vi "FaulhaberV3-Ascii_V1.vi"() -> (1 "searchnames":string[](array[string]), 2 "ID":u32[](array[numeric]), 3 "Faulhaber Objects":T3(array[cluster]))   [LabVIEW 2011] (continued)
7\" dataType=\"0006\" accessType=\"ro\" PDOmapping=\"TPDO\" />\n\t\t\t\t\t</CANopenObject>\n\t\t\t\t\t<CANopenObject index=\"2316\" name=\"Reference encoder\" objectType=\"9\" subNumber=\"8\">\n\t\t\t\t\t\t<CANopenSubObject subIndex=\"00\" name=\"Number of entries\" objectType=\"7\" dataType=\"0005\" accessType=\"ro\" defaultValue=\"9\" PDOmapping=\"no\" />\n\t\t\t\t\t\t<CANopenSubObject subIndex=\"01\" name=\"Operation mode, index polarity\" objectType=\"7\" dataType=\"0006\" lowLimit=\"0\" highLimit=\"0x0107\" accessType=\"rw\" defaultValue=\"0x0\" PDOmapping=\"no\" objFlags=\"00020000\" />\n\t\t\t\t\t\t<CANopenSubObject subIndex=\"02\" name=\"IE resolution\" objectType=\"7\" dataType=\"0007\" lowLimit=\"0\" highLimit=\"4294967295\" accessType=\"rw\" defaultValue=\"2048\" PDOmapping=\"no\" objFlags=\"00020000\" />\n\t\t\t\t\t\t<CANopenSubObject subIndex=\"03\" name=\"Reference encoder position\" objectType=\"7\" dataType=\"0004\" accessType=\"ro\" PDOmapping=\"TPDO\" />\n\t\t\t\t\t\t<CANopenSubObject subIndex=\"04\" name=\"Gain  (numerator/divisor)\" objectType=\"7\" dataType=\"0004\" lowLimit=\"-2147483648\" highLimit=\"2147483647\" accessType=\"rw\" defaultValue=\"0x40004000\" PDOmapping=\"RPDO\" objFlags=\"00020000\" />\n\t\t\t\t\t\t<CANopenSubObject subIndex=\"05\" name=\"RefEnc scaled position\" objectType=\"7\" dataType=\"0004\" lowLimit=\"-2147483648\" highLimit=\"2147483647\" accessType=\"rw\" defaultValue=\"0\" PDOmapping=\"TPDO\" />\n\t\t\t\t\t\t<CANopenSubObject subIndex=\"08\" name=\"Reference encoder act speed\" objectType=\"7\" dataType=\"0004\" accessType=\"ro\" PDOmapping=\"TPDO\" />\n\t\t\t\t\t\t<CANopenSubObject subIndex=\"09\" name=\"Speed filter\" objectType=\"7\" dataType=\"0006\" lowLimit=\"0\" highLimit=\"65535\" accessType=\"rw\" defaultValue=\"10\" PDOmapping=\"TPDO\" objFlags=\"00020000\" />\n\t\t\t\t\t</CANopenObject>\n\t\t\t\t\t<CANopenObject index=\"2317\" name=\"PWM input\" objectType=\"9\" subNumber=\"8\">\n\t\t\t\t\t\t<CANopenSubObject subIndex=\"00\" name=\"Number of entries\" objectType=\"7\" dataType=\"0005\" accessType=\"ro\" defaultValue=\"7\" PDOmapping=\"no\" />\n\t\t\t\t\t\t<CANopenSubObject subIndex=\"01\" name=\"Digital input pin\" objectType=\"7\" dataType=\"0005\" PDOmapping=\"no\" objFlags=\"00020000\" uniqueIDRef=\"UID_PARAM_231701\" />\n\t\t\t\t\t\t<CANopenSubObject subIndex=\"02\" name=\"PWM input frequency\" objectType=\"7\" dataType=\"0007\" accessType=\"ro\" PDOmapping=\"TPDO\" objFlags=\"00020000\" />\n\t\t\t\t\t\t<CANopenSubObject subIndex=\"03\" name=\"Duty cycle raw value\" objectType=\"7\" dataType=\"0003\" accessType=\"ro\" PDOmapping=\"TPDO\" objFlags=\"00020000\" />\n\t\t\t\t\t\t<CANopenSubObject subIndex=\"04\" name=\"Duty cycle  gain (numerator/divisor)\" objectType=\"7\" dataType=\"0007\" lowLimit=\"0\" highLimit=\"4294967295\" accessType=\"rw\" defaultValue=\"0x7FFF8000\" PDOmapping=\"no\" objFlags=\"00020000\" />\n\t\t\t\t\t\t<CANopenSubObject subIndex=\"05\" name=\"Duty cycle offset\" objectType=\"7\" dataType=\"0003\" lowLimit=\"-32768\" highLimit=\"32767\" accessType=\"rw\" defaultValue=\"0\" PDOmapping=\"RPDO\" objFlags=\"00020000\" />\n\t\t\t\t\t\t<CANopenSubObject subIndex=\"06\" name=\"Duty cycle scaled value\" objectType=\"7\" dataType=\"0004\" accessType=\"ro\" PDOmapping=\"TPDO\" objFlags=\"00020000\" />\n\t\t\t\t\t\t<CANopenSubObject subIndex=\"07\" name=\"Resolution as encoder\" objectType=\"7\" dataType=\"0003\" lowLimit=\"-32768\" highLimit=\"32767\" accessType=\"rw\" defaultValue=\"1000\" PDOmapping=\"no\" objFlags=\"00020000\" />\n\t\t\t\t\t</CANopenObject>\n\t\t\t\t\t<CANopenObject index=\"2318\" name=\"Hall configuration\" objectType=\"9\" subNumber=\"6\">\n\t\t\t\t\t\t<CANopenSubObject subIndex=\"00\" name=\"Number of entries\" objectType=\"7\" dataType=\"0005\" accessType=\"ro\" defaultValue=\"5\" PDOmapping=\"no\" />\n\t\t\t\t\t\t<CANopenSubObject subIndex=\"01\" name=\"Hall sensor type\" objectType=\"7\" dataType=\"0005\" highLimit=\"0x83\" accessType=\"ro\" PDOmapping=\"no\" objFlags=\"00030000\" />\n\t\t\t\t\t\t<CANopenSubObject subIndex=\"02\" name=\"Enable adaptation\" objectType=\"7\" dataType=\"0005\" lowLimit=\"0\" highLimit=\"255\" accessType=\"rw\" defaultValue=\"0\" PDOmapping=\"no\" objFlags=\"00020000\" />\n\t\t\t\t\t\t<CANopenSubObject subIndex=\"03\" name=\"Adaptation threshold speed\" objectType=\"7\" dataType=\"0007\" lowLimit=\"0\" highLimit=\"4294967295\" accessType=\"rw\" defaultValue=\"1000\" PDOmapping=\"no\" objFlags=\"00020000\" />\n\t\t\t\t\t\t<CANopenSubObject subIndex=\"04\" name=\"Digital hall settings of Non-Faulhaber motors\" objectType=\"7\" dataType=\"0005\" lowLimit=\"0\" highLimit=\"0x81\" accessType=\"rw\" defaultValue=\"0x0\" PDOmapping=\"no\" objFlags=\"00020000\" />\n\t\t\t\t\t\t<CANopenSubObject subIndex=\"05\" name=\"Hall filter configuration\" objectType=\"7\" dataType=\"0005\" lowLimit=\"0\" highLimit=\"0x03\" accessType=\"rw\" defaultValue=\"0x0\" PDOmapping=\"no\" objFlags=\"00020000\" />\n\t\t\t\t\t</CANopenObject>\n\t\t\t\t\t<CANopenObject index=\"2319\" name=\"Reduction ratio, external position encoder\" objectType=\"8\" subNumber=\"3\">\n\t\t\t\t\t\t<CANopenSubObject subIndex=\"00\" name=\"Number of entries\" objectType=\"7\" dataType=\"0005\" accessType=\"ro\" defaultValue=\"2\" PDOmapping=\"no\" />\n\t\t\t\t\t\t<CANopenSubObject subIndex=\"01\" name=\"Numerator\" objectType=\"7\" dataType=\"0007\" lowLimit=\"1\" highLimit=\"4294967295\" accessType=\"rw\" defaultValue=\"1\" PDOmapping=\"RPDO\" objFlags=\"00020000\" />\n\t\t\t\t\t\t<CANopenSubObject subIndex=\"02\" name=\"Divisor\" objectType=\"7\" dataType=\"0007\" lowLimit=\"1\" highLimit=\"4294967295\" accessType=\"rw\" defaultValue=\"1\" PDOmapping=\"RPDO\" objFlags=\"00020000\" />\n\t\t\t\t\t</CANopenObject>\n\t\t\t\t\t<CANopenObject index=\"231F\" name=\"231F_00\" objectType=\"8\" subNumber=\"16\">\n\t\t\t\t\t\t<CANopenSubObject subIndex=\"00\" name=\"Number of entries\" objectType=\"7\" dataType=\"0005\" accessType=\"ro\" defaultValue=\"15\" PDOmapping=\"no\" objFlags=\"00020003\" />\n\t\t\t\t\t\t<CANopenSubObject subIndex=\"01\" name=\"231F_01\" objectType=\"7\" dataType=\"0003\" accessType=\"ro\" PDOmapping=\"no\" objFlags=\"00020003\" />\n\t\t\t\t\t\t<CANopenSubObject subIndex=\"02\" name=\"231F_02\" objectType=\"7\" dataType=\"0003\" accessType=\"ro\" PDOmapping=\"no\" objFlags=\"00020003\" />\n\t\t\t\t\t\t<CANopenSubObject subIndex=\"03\" name=\"231F_03\" objectType=\"7\" dataType=\"0003\" accessType=\"ro\" PDOmapping=\"no\" objFlags=\"00020003\" />\n\t\t\t\t\t\t<CANopenSubObject subIndex=\"04\" name=\"231F_04\" objectType=\"7\" dataType=\"0003\" accessType=\"ro\" PDOmapping=\"no\" objFlags=\"00020003\" />\n\t\t\t\t\t\t<CANopenSubObject subIndex=\"05\" name=\"231F_05\" objectType=\"7\" dataType=\"0003\" accessType=\"ro\" PDOmapping=\"no\" objFlags=\"00020003\" />\n\t\t\t\t\t\t<CANopenSubObject subIndex=\"06\" name=\"231F_06\" objectType=\"7\" dataType=\"0003\" accessType=\"ro\" PDOmapping=\"no\" objFlags=\"00020003\" />\n\t\t\t\t\t\t<CANopenSubObject subIndex=\"07\" name=\"231F_07\" objectType=\"7\" dataType=\"0003\" accessType=\"ro\" PDOmapping=\"no\" objFlags=\"00020003\" />\n\t\t\t\t\t\t<CANopenSubObject subIndex=\"08\" name=\"231F_08\" objectType=\"7\" dataType=\"0003\" accessType=\"ro\" PDOmapping=\"no\" objFlags=\"00020003\" />\n\t\t\t\t\t\t<CANopenSubObject subIndex=\"09\" name=\"231F_09\" objectType=\"7\" dataType=\"0003\" accessType=\"ro\" PDOmapping=\"no\" objFlags=\"00020003\" />\n\t\t\t\t\t\t<CANopenSubObject subIndex=\"0A\" name=\"231F_0A\" objectType=\"7\" dataType=\"0003\" accessType=\"ro\" PDOmapping=\"no\" objFlags=\"00020003\" />\n\t\t\t\t\t\t<CANopenSubObject subIndex=\"0B\" name=\"231F_0B\" objectType=\"7\" dataType=\"0003\" accessType=\"ro\" PDOmapping=\"no\" objFlags=\"00020003\" />\n\t\t\t\t\t\t<CANopenSubObject subIndex=\"0C\" name=\"231F_0C\" objectType=\"7\" dataType=\"0003\" accessType=\"ro\" PDOmapping=\"no\" objFlags=\"00020003\" />\n\t\t\t\t\t\t<CANopenSubObject subIndex=\"0D\" name=\"231F_0D\" objectType=\"7\" dataType=\"0003\" accessType=\"ro\" PDOmapping=\"no\" objFlags=\"00020003\" />\n\t\t\t\t\t\t<CANopenSubObject subIndex=\"0E\" name=\"231F_0E\" objectType=\"7\" dataType=\"0003\" accessType=\"ro\" PDOmapping=\"no\" objFlags=\"00020003\" />\n\t\t\t\t\t\t<CANopenSubObject subIndex=\"0F\" name=\"231F_0F\" objectType=\"7\" dataType=\"0003\" accessType=\"ro\" PDOmapping=\"no\" objFlags=\"00020003\" />\n\t\t\t\t\t</CANopenObject>\n\t\t\t\t\t<CANopenObject index=\"2320\" name=\"Faulhaber error register\" objectType=\"7\" dataType=\"0006\" accessType=\"ro\" PDOmapping=\"TPDO\" />\n\t\t\t\t\t<CANopenObject index=\"2321\" name=\"Error mask\" objectType=\"8\" subNumber=\"8\">\n\t\t\t\t\t\t<CANopenSubObject subIndex=\"00\" name=\"Number of entries\" objectType=\"7\" dataType=\"0005\" accessType=\"ro\" defaultValue=\"7\" PDOmapping=\"no\" />\n\t\t\t\t\t\t<CANopenSubObject subIndex=\"01\" name=\"EMCY mask\" objectType=\"7\" dataType=\"0006\" lowLimit=\"0\" highLimit=\"65535\" accessType=\"rw\" defaultValue=\"0xFFFF\" PDOmapping=\"RPDO\" objFlags=\"00020000\" />\n\t\t\t\t\t\t<CANopenSubObject subIndex=\"02\" name=\"Fault mask\" objectType=\"7\" dataType=\"0006\" lowLimit=\"0\" highLimit=\"0xBFD3\" accessType=\"rw\" defaultValue=\"0x0000\" PDOmapping=\"RPDO\" objFlags=\"00020000\" />\n\t\t\t\t\t\t<CANopenSubObject subIndex=\"03\" name=\"Error out mask\" objectType=\"7\" dataType=\"0006\" lowLimit=\"0\" highLimit=\"65535\" accessType=\"rw\" defaultValue=\"0x0000\" PDOmapping=\"RPDO\" objFlags=\"00020000\" />\n\t\t\t\t\t\t<CANopenSubObject subIndex=\"04\" name=\"Disable voltage mask manufacturer\" objectType=\"7\" dataType=\"0006\" accessType=\"ro\" defaultValue=\"0x402C\" PDOmapping=\"no\" objFlags=\"00030000\" />\n\t\t\t\t\t\t<CANopenSubObject subIndex=\"05\" name=\"Disable voltage mask user\" objectType=\"7\" dataType=\"0006\" lowLimit=\"0\" highLimit=\"0xBFD3\" accessType=\"rw\" defaultValue=\"0x0000\" PDOmapping=\"RPDO\" objFlags=\"00020000\" />\n\t\t\t\t\t\t<CANopenSubObject subIndex=\"06\" name=\"Quick stop mask\" objectType=\"7\" dataType=\"0006\" lowLimit=\"0\" highLimit=\"0xBFD3\" accessType=\"rw\" defaultValue=\"0x0000\" PDOmapping=\"RPDO\" objFlags=\"00020000\" />\n\t\t\t\t\t\t<CANopenSubObject subIndex=\"07\" name=\"Error bit mask\" objectType=\"7\" dataType=\"0006\" lowLimit=\"0\" highLimit=\"65535\" accessType=\"rw\" defaultValue=\"0x0000\" PDOmapping=\"RPDO\" objFlags=\"00020000\" />\n\t\t\t\t\t</CANopenObject>\n\t\t\t\t\t<CANopenObject index=\"2322\" name=\"Error codes\" objectType=\"8\" subNumber=\"2\">\n\t\t\t\t\t\t<CANopenSubObject subIndex=\"00\" name=\"Number of entries\" objectType=\"7\" dataType=\"0005\" accessType=\"ro\" defaultValue=\"1\" PDOmapping=\"no\" />\n\t\t\t\t\t\t<CANopenSubObject subIndex=\"01\" name=\"ScriptingError\" objectType=\"7\" dataType=\"0006\" accessType=\"ro\" defaultValue=\"0\" PDOmapping=\"TPDO\" />\n\t\t\t\t\t</CANopenObject>\n\t\t\t\t\t<CANopenObject index=\"2324\" name=\"Device status\" objectType=\"9\" subNumber=\"10\">\n\t\t\t\t\t\t<CANopenSubObject subIndex=\"00\" name=\"Number of entries\" objectType=\"7\" dataType=\"0005\" accessType=\"ro\" defaultValue=\"9\" PDOmapping=\"no\" />\n\t\t\t\t\t\t<CANopenSubObject subIndex=\"01\" name=\"Device status word\" objectType=\"7\" dataType=\"0007\" lowLimit=\"0x0\" accessType=\"ro\" PDOmapping=\"TPDO\" />\n\t\t\t\t\t\t<CANopenSubObject subIndex=\"02\" name=\"Limit check delay time\" objectType=\"7\" dataType=\"0006\" lowLimit=\"0\" highLimit=\"65535\" accessType=\"rw\" defaultValue=\"10\" PDOmapping=\"RPDO\" objFlags=\"00020000\" />\n\t\t\t\t\t\t<CANopenSubObject subIndex=\"03\" name=\"Reserved 3\" objectType=\"7\" dataType=\"0005\" accessType=\"ro\" PDOmapping=\"TPDO\" objFlags=\"00020003\" />\n\t\t\t\t\t\t<CANopenSubObject subIndex=\"04\" name=\"Reserved 4\" objectType=\"7\" dataType=\"0003\" accessType=\"ro\" PDOmapping=\"TPDO\" objFlags=\"00020003\" />\n\t\t\t\t\t\t<CANopenSubObject subIndex=\"05\" name=\"Reserved 5\" objectType=\"7\" dataType=\"0003\" accessType=\"ro\" PDOmapping=\"TPDO\" objFlags=\"00020003\" />\n\t\t\t\t\t\t<CANopenSubObject subIndex=\"06\" name=\"Reserved 6\" objectType=\"7\" dataType=\"0004\" accessType=\"ro\" PDOmapping=\"TPDO\" objFlags=\"00020003\" />\n\t\t\t\t\t\t<CANopenSubObject subIndex=\"07\" name=\"Reserved 7\" objectType=\"7\" dataType=\"0004\" accessType=\"ro\" PDOmapping=\"TPDO\" objFlags=\"00020003\" />\n\t\t\t\t\t\t<CANopenSubObject subIndex=\"08\" name=\"Reserved 8\" objectType=\"7\" dataType=\"0005\" lowLimit=\"0\" highLimit=\"255\" accessType=\"wo\" PDOmapping=\"TPDO\" objFlags=\"00020003\" />\n\t\t\t\t\t\t<CANopenSubObject subIndex=\"09\" name=\"Reserved 9\" objectType=\"7\" dataType=\"0005\" lowLimit=\"0\" highLimit=\"255\" accessType=\"wo\" PDOmapping=\"TPDO\" objFlags=\"00020003\" />\n\t\t\t\t\t</CANopenObject>\n\t\t\t\t\t<CANopenObject index=\"2325\" name=\"Voltage monitor\" objectType=\"9\" subNumber=\"8\">\n\t\t\t\t\t\t<CANopenSubObject subIndex=\"00\" name=\"Number of entries\" objectType=\"7\" dataType=\"0005\" accessType=\"ro\" defaultValue=\"7\" PDOmapping=\"no\" />\n\t\t\t\t\t\t<CANopenSubObject subIndex=\"01\" name=\"Device supply lower threshold\" objectType=\"7\" dataType=\"0006\" accessType=\"ro\" PDOmapping=\"TPDO\" objFlags=\"00030000\" />\n\t\t\t\t\t\t<CANopenSubObject subIndex=\"02\" name=\"Motor supply lower threshold\" objectType=\"7\" dataType=\"0006\" lowLimit=\"0\" highLimit=\"65535\" accessType=\"rw\" PDOmapping=\"TPDO\" objFlags=\"00020000\" />\n\t\t\t\t\t\t<CANopenSubObject subIndex=\"03\" name=\"Motor supply max threshold\" objectType=\"7\" dataType=\"0006\" accessType=\"ro\" PDOmapping=\"TPDO\" objFlags=\"00030000\" />\n\t\t\t\t\t\t<CANopenSubObject subIndex=\"04\" name=\"Motor supply upper threshold\" objectType=\"7\" dataType=\"0006\" lowLimit=\"0\" highLimit=\"65535\" accessType=\"rw\" PDOmapping=\"TPDO\" objFlags=\"00020000\" />\n\t\t\t\t\t\t<CANopenSubObject subIndex=\"05\" name=\"Voltage error delay time\" objectType=\"7\" dataType=\"0006\" lowLimit=\"0\" highLimit=\"65535\" accessType=\"rw\" defaultValue=\"200\" PDOmapping=\"TPDO\" objFlags=\"00020000\" />\n\t\t\t\t\t\t<CANopenSubObject subIndex=\"06\" name=\"Device supply voltage\" objectType=\"7\" dataType=\"0006\" accessType=\"ro\" PDOmapping=\"TPDO\" />\n\t\t\t\t\t\t<CANopenSubObject subIndex=\"07\" name=\"Motor supply voltage\" objectType=\"7\" dataType=\"0006\" accessType=\"ro\" PDOmapping=\"TPDO\" />\n\t\t\t\t\t</CANopenObject>\n\t\t\t\t\t<CANopenObject index=\"2326\" name=\"Device temperature\" objectType=\"9\" subNumber=\"12\">\n\t\t\t\t\t\t<CANopenSubObject subIndex=\"00\" name=\"Number of entries\" objectType=\"7\" dataType=\"0005\" accessType=\"ro\" defaultValue=\"11\" PDOmapping=\"no\" />\n\t\t\t\t\t\t<CANopenSubObject subIndex=\"01\" name=\"CPU temperature\" objectType=\"7\" dataType=\"0003\" accessType=\"ro\" PDOmapping=\"TPDO\" />\n\t\t\t\t\t\t<CANopenSubObject subIndex=\"02\" name=\"Power stage temperature\" objectType=\"7\" dataType=\"0003\" accessType=\"ro\" PDOmapping=\"TPDO\" />\n\t\t\t\t\t\t<CANopenSubObject subIndex=\"03\" name=\"Winding temperature\" objectType=\"7\" dataType=\"0003\" accessType=\"ro\" PDOmapping=\"TPDO\" />\n\t\t\t\t\t\t<CANopenSubObject subIndex=\"04\" name=\"CPU temperature shutdown threshold\" objectType=\"7\" dataType=\"0003\" accessType=\"ro\" PDOmapping=\"no\" objFlags=\"00030000\" />\n\t\t\t\t\t\t<CANopenSubObject subIndex=\"05\" name=\"CPU temperature warning threshold\" objectType=\"7\" dataType=\"0003\" accessType=\"ro\" PDOmapping=\"no\" objFlags=\"00030000\" />\n\t\t\t\t\t\t<CANopenSubObject subIndex=\"06\" name=\"Power stage temperature shutdown threshold\" objectType=\"7\" dataType=\"0003\" accessType=\"ro\" PDOmapping=\"no\" objFlags=\"00030000\" />\n\t\t\t\t\t\t<CANopenSubObject subIndex=\"07\" name=\"Power stage temperature warning threshold\" objectType=\"7\" dataType=\"0003\" accessType=\"ro\" PDOmapping=\"no\" objFlags=\"00030000\" />\n\t\t\t\t\t\t<CANopenSubObject subIndex=\"08\" name=\"Winding temperature shutdown threshold\" objectType=\"7\" dataType=\"0003\" lowLimit=\"-32768\" highLimit=\"32767\" accessType=\"rw\" PDOmapping=\"no\" objFlags=\"00020000\" />\n\t\t\t\t\t\t<CANopenSubObject subIndex=\"09\" name=\"Winding temperature warning threshold\" objectType=\"7\" dataType=\"0003\" lowLimit=\"-32768\" highLimit=\"32767\" accessType=\"rw\" PDOmapping=\"no\" objFlags=\"00020000\" />\n\t\t\t\t\t\t<CANopenSubObject subIndex=\"0A\" name=\"Motor NTC temperature\" objectType=\"7\" dataType=\"0003\" accessType=\"ro\" PDOmapping=\"TPDO\" />\n\t\t\t\t\t\t<CANopenSubObject subIndex=\"0B\" name=\"Motor NTC enable\" objectType=\"7\" dataType=\"0003\" lowLimit=\"0\" highLimit=\"1\" accessType=\"ro\" defaultValue=\"1\" PDOmapping=\"no\" objFlags=\"00030000\" />\n\t\t\t\t\t</CANopenObject>\n\t\t\t\t\t<CANopenObject index=\"2327\" name=\"Device data\" objectType=\"9\" subNumber=\"4\">\n\t\t\t\t\t\t<CANopenSubObject subIndex=\"00\" name=\"Number of entries\" objectType=\"7\" dataType=\"0005\" accessType=\"ro\" defaultValue=\"3\" PDOmapping=\"no\" />\n\t\t\t\t\t\t<CANopenSubObject subIndex=\"01\" name=\"Device nominal current\" objectType=\"7\" dataType=\"0006\" lowLimit=\"1000\" highLimit=\"5000\" accessType=\"ro\" PDOmapping=\"no\" objFlags=\"00030000\" />\n\t\t\t\t\t\t<CANopenSubObject subIndex=\"02\" name=\"Device peak current\" objectType=\"7\" dataType=\"0006\" accessType=\"ro\" PDOmapping=\"no\" objFlags=\"00030000\" />\n\t\t\t\t\t\t<CANopenSubObject subIndex=\"03\" name=\"Device nominal voltage\" objectType=\"7\" dataType=\"0006\" accessType=\"ro\" PDOmapping=\"no\" objFlags=\"00030000\" />\n\t\t\t\t\t</CANopenObject>\n\t\t\t\t\t<CANopenObject index=\"2328\" name=\"Device data for thermal model\" objectType=\"9\" subNumber=\"10\">\n\t\t\t\t\t\t<CANopenSubObject subIndex=\"00\" name=\"Number of entries\" objectType=\"7\" dataType=\"0005\" accessType=\"ro\" defaultValue=\"9\" PDOmapping=\"no\" />\n\t\t\t\t\t\t<CANopenSubObject subIndex=\"01\" name=\"Controller type\" objectType=\"7\" dataType=\"0005\" PDOmapping=\"no\" objFlags=\"00030000\" uniqueIDRef=\"UID_PARAM_232801\" />\n\t\t\t\t\t\t<CANopenSubObject subIndex=\"02\" name=\"Power stage Rdson\" objectType=\"7\" dataType=\"0005\" accessType=\"ro\" PDOmapping=\"no\" objFlags=\"00030000\" />\n\t\t\t\t\t\t<CANopenSubObject subIndex=\"03\" name=\"Power stage LossFactor\" objectType=\"7\" dataType=\"0006\" accessType=\"ro\" PDOmapping=\"no\" objFlags=\"00030000\" />\n\t\t\t\t\t\t<CANopenSubObject subIndex=\"04\" name=\"Power stage Rth1\" objectType=\"7\" dataType=\"0006\" accessType=\"ro\" PDOmapping=\"no\" objFlags=\"00030000\" />\n\t\t\t\t\t\t<CANopenSubObject subIndex=\"05\" name=\"Power stage Time Constant 1\" objectType=\"7\" dataType=\"0006\" accessType=\"ro\" PDOmapping=\"no\" objFlags=\"00030000\" />\n\t\t\t\t\t\t<CANopenSubObject subIndex=\"06\" name=\"Power stage Rth2\" objectType=\"7\" dataType=\"0006\" accessType=\"ro\" PDOmapping=\"no\" objFlags=\"00030000\" />\n\t\t\t\t\t\t<CANopenSubObject subIndex=\"07\" name=\"Power stage Time Constant 2\" objectType=\"7\" dataType=\"0006\" accessType=\"ro\" PDOmapping=\"no\" objFlags=\"00030000\" />\n\t\t\t\t\t\t<CANopenSubObject subIndex=\"08\" name=\"Power stage Rth3\" objectType=\"7\" dataType=\"0006\" accessType=\"ro\" PDOmapping=\"no\" objFlags=\"00030000\" />\n\t\t\t\t\t\t<CANopenSubObject subIndex=\"09\" name=\"Power stage Rth4\" objectType=\"7\" dataType=\"0006\" accessType=\"ro\" PDOmapping=\"no\" objFlags=\"00030000\" />\n\t\t\t\t\t</CANopenObject>\n\t\t\t\t\t<CANopenObject index=\"2329\" name=\"Motor and application data for motor control\" objectType=\"9\" subNumber=\"19\">\n\t\t\t\t\t\t<CANopenSubObject subIndex=\"00\" name=\"Number of entries\" objectType=\"7\" dataType=\"0005\" accessType=\"ro\" defaultValue=\"18\" PDOmapping=\"no\" />\n\t\t\t\t\t\t<CANopenSubObject subIndex=\"01\" name=\"Rated current\" objectType=\"7\" dataType=\"0006\" lowLimit=\"0\" highLimit=\"65535\" accessType=\"rw\" PDOmapping=\"no\" objFlags=\"00020000\" />\n\t\t\t\t\t\t<CANopenSubObject subIndex=\"02\" name=\"Continous current\" objectType=\"7\" dataType=\"0006\" lowLimit=\"0\" highLimit=\"65535\" accessType=\"rw\" PDOmapping=\"no\" objFlags=\"00020000\" />\n\t\t\t\t\t\t<CANopenSubObject subIndex=\"03\" name=\"Peak current\" objectType=\"7\" dataType=\"0006\" lowLimit=\"0\" highLimit=\"65535\" accessType=\"rw\" PDOmapping=\"no\" objFlags=\"00020000\" />\n\t\t\t\t\t\t<CANopenSubObject subIndex=\"04\" name=\"Torque constant / Force constant\" objectType=\"7\" dataType=\"0007\" lowLimit=\"0\" highLimit=\"3500000\" accessType=\"rw\" PDOmapping=\"no\" objFlags=\"00020000\" />\n\t\t\t\t\t\t<CANopenSubObject subIndex=\"05\" name=\"Terminal inductance\" objectType=\"7\" dataType=\"0007\" lowLimit=\"0\" highLimit=\"200000\" accessType=\"rw\" PDOmapping=\"no\" objFlags=\"00020000\" />\n\t\t\t\t\t\t<CANopenSubObject subIndex=\"06\" name=\"Inductance Ld\" objectType=\"7\" dataType=\"0007\" lowLimit=\"0\" highLimit=\"200000\" accessType=\"rw\" PDOmapping=\"no\" objFlags=\"00020000\" />\n\t\t\t\t\t\t<CANopenSubObject subIndex=\"07\" name=\"Number of pole pairs\" objectType=\"7\" dataType=\"0005\" accessType=\"ro\" PDOmapping=\"no\" objFlags=\"00030000\" />\n\t\t\t\t\t\t<CANopenSubObject subIndex=\"08\" name=\"Phase angle offset\" objectType=\"7\" dataType=\"0003\" lowLimit=\"-32768\" highLimit=\"32767\" accessType=\"rw\" PDOmapping=\"no\" objFlags=\"00020001\" />\n\t\t\t\t\t\t<CANopenSubObject subIndex=\"09\" name=\"Rotor inertia / Rod weight\" objectType=\"7\" dataType=\"0007\" lowLimit=\"0\" highLimit=\"4294967295\" accessType=\"rw\" PDOmapping=\"no\" objFlags=\"00020000\" />\n\t\t\t\t\t\t<CANopenSubObject subIndex=\"0A\" name=\"Load inertia / Load mass\" objectType=\"7\" dataType=\"0007\" lowLimit=\"0\" highLimit=\"4294967295\" accessType=\"rw\" PDOmapping=\"RPDO\" objFlags=\"00020000\" />\n\t\t\t\t\t\t<CANopenSubObject subIndex=\"0B\" name=\"Motor type\" objectType=\"7\" dataType=\"0005\" PDOmapping=\"no\" objFlags=\"00030000\" uniqueIDRef=\"UID_PARAM_23290B\" />\n\t\t\t\t\t\t<CANopenSubObject subIndex=\"0C\" name=\"Magnetic pitch of linear motor\" objectType=\"7\" dataType=\"0005\" lowLimit=\"0\" highLimit=\"60\" accessType=\"rw\" PDOmapping=\"no\" objFlags=\"00020000\" />\n\t\t\t\t\t\t<CANopenSubObject subIndex=\"0D\" name=\"Filter phase inductance\" objectType=\"7\" dataType=\"0005\" lowLimit=\"0\" highLimit=\"255\" accessType=\"rw\" PDOmapping=\"no\" objFlags=\"00020000\" />\n\t\t\t\t\t\t<CANopenSubObject subIndex=\"0E\" name=\"Factor speed constant\" objectType=\"7\" dataType=\"0006\" lowLimit=\"750\" highLimit=\"1250\" accessType=\"rw\" PDOmapping=\"no\" objFlags=\"00020001\" />\n\t\t\t\t\t\t<CANopenSubObject subIndex=\"0F\" name=\"Steps per turn\" objectType=\"7\" dataType=\"0006\" lowLimit=\"0\" highLimit=\"65535\" accessType=\"rw\" defaultValue=\"24\" PDOmapping=\"no\" objFlags=\"00020003\" />\n\t\t\t\t\t\t<CANopenSubObject subIndex=\"10\" name=\"Stepper interpolation factor\" objectType=\"7\" dataType=\"0006\" lowLimit=\"0\" highLimit=\"65535\" accessType=\"rw\" defaultValue=\"512\" PDOmapping=\"no\" objFlags=\"00020003\" />\n\t\t\t\t\t\t<CANopenSubObject subIndex=\"11\" name=\"Stepper current reduction at n=0\" objectType=\"7\" dataType=\"0005\" lowLimit=\"0\" highLimit=\"100\" accessType=\"rw\" defaultValue=\"60\" PDOmapping=\"no\" objFlags=\"00020003\" />\n\t\t\t\t\t\t<CANopenSubObject subIndex=\"12\" name=\"Current holding time at n=0\" objectType=\"7\" dataType=\"0006\" lowLimit=\"0\" highLimit=\"65535\" accessType=\"rw\" defaultValue=\"200\" PDOmapping=\"no\" objFlags=\"00020003\" />\n\t\t\t\t\t</CANopenObject>\n\t\t\t\t\t<CANopenObject index=\"232A\" name=\"Motor and application data for thermal motor model\" objectType=\"9\" subNumber=\"11\">\n\t\t\t\t\t\t<CANopenSubObject subIndex=\"00\" name=\"Number of entries\" objectType=\"7\" dataType=\"0005\" accessType=\"ro\" defaultValue=\"10\" PDOmapping=\"no\" />\n\t\t\t\t\t\t<CANopenSubObject subIndex=\"01\" name=\"Terminal resistance\" objectType=\"7\" dataType=\"0007\" lowLimit=\"0\" highLimit=\"4294967295\" accessType=\"rw\" PDOmapping=\"no\" objFlags=\"00020000\" />\n\t\t\t\t\t\t<CANopenSubObject subIndex=\"02\" name=\"Friction\" objectType=\"7\" dataType=\"0007\" lowLimit=\"0\" highLimit=\"4294967295\" accessType=\"rw\" PDOmapping=\"no\" objFlags=\"00020000\" />\n\t\t\t\t\t\t<CANopenSubObject subIndex=\"03\" name=\"Friction,dynamic\" objectType=\"7\" dataType=\"0007\" lowLimit=\"0\" highLimit=\"4294967295\" accessType=\"rw\" PDOmapping=\"no\" objFlags=\"00020000\" />\n\t\t\t\t\t\t<CANopenSubObject subIndex=\"04\" name=\"Thermal resistance 1\" objectType=\"7\" dataType=\"0006\" lowLimit=\"0\" highLimit=\"65535\" accessType=\"rw\" PDOmapping=\"no\" objFlags=\"00020000\" />\n\t\t\t\t\t\t<CANopenSubObject subIndex=\"05\" name=\"Thermal resistance 2\" objectType=\"7\" dataType=\"0007\" lowLimit=\"0\" highLimit=\"4294967295\" accessType=\"rw\" PDOmapping=\"no\" objFlags=\"00020000\" />\n\t\t\t\t\t\t<CANopenSubObject subIndex=\"06\" name=\"Thermal time constant 1\" objectType=\"7\" dataType=\"0006\" lowLimit=\"0\" highLimit=\"65535\" accessType=\"rw\" PDOmapping=\"no\" objFlags=\"00020000\" />\n\t\t\t\t\t\t<CANopenSubObject subIndex=\"07\" name=\"Thermal time constant 2\" objectType=\"7\" dataType=\"0006\" lowLimit=\"0\" highLimit=\"65535\" accessType=\"rw\" PDOmapping=\"no\" objFlags=\"00020000\" />\n\t\t\t\t\t\t<CANopenSubObject subIndex=\"08\" name=\"Ambient temperature\" objectType=\"7\" dataType=\"0005\" lowLimit=\"0\" highLimit=\"255\" accessType=\"rw\" defaultValue=\"22\" PDOmapping=\"no\" objFlags=\"00020000\" />\n\t\t\t\t\t\t<CANopenSubObject subIndex=\"09\" name=\"Reduction of thermal resistance 2\" objectType=\"7\" dataType=\"0005\" lowLimit=\"0\" highLimit=\"99\" accessType=\"rw\" defaultValue=\"25\" PDOmapping=\"no\" objFlags=\"00020000\" />\n\t\t\t\t\t\t<CANopenSubObject subIndex=\"0A\" name=\"Selection of thermal model\" objectType=\"7\" dataType=\"0005\" lowLimit=\"0\" highLimit=\"2\" accessType=\"rw\" defaultValue=\"0\" PDOmapping=\"no\" objFlags=\"00020000\" />\n\t\t\t\t\t</CANopenObject>\n\t\t\t\t\t<CANopenObject index=\"232B\" name=\"Motor alignment parameters\" objectType=\"9\" subNumber=\"6\">\n\t\t\t\t\t\t<CANopenSubObject subIndex=\"00\" name=\"Number of entries\" objectType=\"7\" dataType=\"0005\" accessType=\"ro\" defaultValue=\"5\" PDOmapping=\"no\" />\n\t\t\t\t\t\t<CANopenSubObject subIndex=\"01\" name=\"Setup time\" objectType=\"7\" dataType=\"0006\" lowLimit=\"0\" highLimit=\"65535\" accessType=\"rw\" defaultValue=\"5\" PDOmapping=\"no\" objFlags=\"00020000\" />\n\t\t\t\t\t\t<CANopenSubObject subIndex=\"02\" name=\"Delta time step 1\" objectType=\"7\" dataType=\"0006\" lowLimit=\"0\" highLimit=\"65535\" accessType=\"rw\" defaultValue=\"250\" PDOmapping=\"no\" objFlags=\"00020000\" />\n\t\t\t\t\t\t<CANopenSubObject subIndex=\"03\" name=\"Delta time step 2\" objectType=\"7\" dataType=\"0006\" lowLimit=\"0\" highLimit=\"65535\" accessType=\"rw\" defaultValue=\"250\" PDOmapping=\"no\" objFlags=\"00020000\" />\n\t\t\t\t\t\t<CANopenSubObject subIndex=\"04\" name=\"Delta time step 3\" objectType=\"7\" dataType=\"0006\" lowLimit=\"0\" highLimit=\"65535\" accessType=\"rw\" defaultValue=\"250\" PDOmapping=\"no\" objFlags=\"00020000\" />\n\t\t\t\t\t\t<CANopenSubObject subIndex=\"05\" name=\"Delta postion tolerance\" objectType=\"7\" dataType=\"0006\" lowLimit=\"0\" highLimit=\"65535\" accessType=\"rw\" defaultValue=\"4096\" PDOmapping=\"no\" objFlags=\"00020000\" />\n\t\t\t\t\t</CANopenObject>\n\t\t\t\t\t<CANopenObject index=\"232C\" name=\"Motor alignment results\" objectType=\"9\" subNumber=\"4\">\n\t\t\t\t\t\t<CANopenSubObject subIndex=\"00\" name=\"Number of entries\" objectType=\"7\" dataType=\"0005\" accessType=\"ro\" defaultValue=\"3\" PDOmapping=\"no\" />\n\t\t\t\t\t\t<CANopenSubObject subIndex=\"01\" name=\"Position A1\" objectType=\"7\" dataType=\"0006\" accessType=\"ro\" PDOmapping=\"no\" objFlags=\"00020003\" />\n\t\t\t\t\t\t<CANopenSubObject subIndex=\"02\" name=\"Position B\" objectType=\"7\" dataType=\"0006\" accessType=\"ro\" PDOmapping=\"no\" objFlags=\"00020003\" />\n\t\t\t\t\t\t<CANopenSubObject subIndex=\"03\" name=\"Position A2\" objectType=\"7\" dataType=\"0006\" accessType=\"ro\" PDOmapping=\"no\" objFlags=\"00020003\" />\n\t\t\t\t\t</CANopenObject>\n\t\t\t\t\t<CANopenObject index=\"2330\" name=\"Switch position for actual values \" objectType=\"8\" subNumber=\"4\">\n\t\t\t\t\t\t<CANopenSubObject subIndex=\"00\" name=\"Number of entries\" objectType=\"7\" dataType=\"0005\" accessType=\"ro\" defaultValue=\"3\" PDOmapping=\"no\" />\n\t\t\t\t\t\t<CANopenSubObject subIndex=\"01\" name=\"Actual commutation angle source\" objectType=\"7\" dataType=\"0005\" PDOmapping=\"RPDO\" objFlags=\"00020000\" uniqueIDRef=\"UID_PARAM_233001\" />\n\t\t\t\t\t\t<CANopenSubObject subIndex=\"02\" name=\"Actual velocity source\" objectType=\"7\" dataType=\"0005\" PDOmapping=\"RPDO\" objFlags=\"00020000\" uniqueIDRef=\"UID_PARAM_233002\" />\n\t\t\t\t\t\t<CANopenSubObject subIndex=\"03\" name=\"Actual position source\" objectType=\"7\" dataType=\"0005\" PDOmapping=\"RPDO\" objFlags=\"00020000\" uniqueIDRef=\"UID_PARAM_233003\" />\n\t\t\t\t\t</CANopenObject>\n\t\t\t\t\t<CANopenObject index=\"2331\" name=\"Discrete sources\" objectType=\"8\" subNumber=\"5\">\n\t\t\t\t\t\t<CANopenSubObject subIndex=\"00\" name=\"Number of entries\" objectType=\"7\" dataType=\"0005\" accessType=\"ro\" defaultValue=\"4\" PDOmapping=\"no\" />\n\t\t\t\t\t\t<CANopenSubObject subIndex=\"01\" name=\"Target voltage source\" objectType=\"7\" dataType=\"0005\" PDOmapping=\"RPDO\" objFlags=\"00020000\" uniqueIDRef=\"UID_PARAM_233101\" />\n\t\t\t\t\t\t<CANopenSubObject subIndex=\"02\" name=\"Target current source\" objectType=\"7\" dataType=\"0005\" PDOmapping=\"RPDO\" objFlags=\"00020000\" uniqueIDRef=\"UID_PARAM_233102\" />\n\t\t\t\t\t\t<CANopenSubObject subIndex=\"03\" name=\"Target velocity source\" objectType=\"7\" dataType=\"0005\" PDOmapping=\"RPDO\" objFlags=\"00020000\" uniqueIDRef=\"UID_PARAM_233103\" />\n\t\t\t\t\t\t<CANopenSubObject subIndex=\"04\" name=\"Target position source\" objectType=\"7\" dataType=\"0005\" PDOmapping=\"RPDO\" objFlags=\"00020000\" uniqueIDRef=\"UID_PARAM_233104\" />\n\t\t\t\t\t</CANopenObject>\n\t\t\t\t\t<CANopenObject index=\"2332\" name=\"Cyclic mode interpolation rate \" objectType=\"7\" dataType=\"0006\" lowLimit=\"1\" highLimit=\"65535\" accessType=\"rw\" defaultValue=\"1\" PDOmapping=\"RPDO\" objFlags=\"00020000\" />\n\t\t\t\t\t<CANopenObject index=\"233A\" name=\"Manufacturer specified bits\" objectType=\"8\" subNumber=\"3\">\n\t\t\t\t\t\t<CANopenSubObject subIndex=\"00\" name=\"Number of entries\" objectType=\"7\" dataType=\"0005\" accessType=\"ro\" defaultValue=\"2\" PDOmapping=\"no\" />\n\t\t\t\t\t\t<CANopenSubObject subIndex=\"01\" name=\"Bit mask for bit 14\" objectType=\"7\" dataType=\"0007\" lowLimit=\"0\" highLimit=\"4294967295\" accessType=\"rw\" defaultValue=\"0x0\" PDOmapping=\"no\" objFlags=\"00020000\" />\n\t\t\t\t\t\t<CANopenSubObject subIndex=\"02\" name=\"Bit mask for bit 15\" objectType=\"7\" dataType=\"0007\" lowLimit=\"0\" highLimit=\"4294967295\" accessType=\"rw\" defaultValue=\"0x0\" PDOmapping=\"no\" objFlags=\"00020000\" />\n\t\t\t\t\t</CANopenObject>\n\t\t\t\t\t<CANopenObject index=\"233E\" name=\"Selection of controller scaling\" objectType=\"7\" dataType=\"0005\" lowLimit=\"0\" highLimit=\"255\" accessType=\"rw\" defaultValue=\"0x00\" PDOmapping=\"no\" objFlags=\"00020000\" />\n\t\t\t\t\t<CANopenObject index=\"233F\" name=\"Operation mode options\" objectType=\"7\" dataType=\"0006\" lowLimit=\"0x0\" highLimit=\"0x80FF\" accessType=\"rw\" PDOmapping=\"no\" objFlags=\"00020000\" />\n\t\t\t\t\t<CANopenObject index=\"2340\" name=\"General parameters\" objectType=\"9\" subNumber=\"10\">\n\t\t\t\t\t\t<CANopenSubObject subIndex=\"00\" name=\"Number of entries\" objectType=\"7\" dataType=\"0005\" accessType=\"ro\" defaultValue=\"9\" PDOmapping=\"no\" />\n\t\t\t\t\t\t<CANopenSubObject subIndex=\"01\" name=\"Commutation type\" objectType=\"7\" dataType=\"0005\" PDOmapping=\"no\" objFlags=\"00020000\" uniqueIDRef=\"UID_PARAM_234001\" />\n\t\t\t\t\t\t<CANopenSubObject subIndex=\"02\" name=\"Motor output voltage DC\" objectType=\"7\" dataType=\"0003\" lowLimit=\"-32768\" highLimit=\"32767\" accessType=\"rw\" defaultValue=\"0\" PDOmapping=\"TPDO\" />\n\t\t\t\t\t\t<CANopenSubObject subIndex=\"03\" name=\"Motor output voltage BL block\" objectType=\"7\" dataType=\"0003\" lowLimit=\"-32768\" highLimit=\"32767\" accessType=\"rw\" defaultValue=\"0\" PDOmapping=\"TPDO\" />\n\t\t\t\t\t\t<CANopenSubObject subIndex=\"04\" name=\"Motor output voltage Xd\" objectType=\"7\" dataType=\"0003\" lowLimit=\"-32768\" highLimit=\"32767\" accessType=\"rw\" defaultValue=\"0\" PDOmapping=\"TPDO\" />\n\t\t\t\t\t\t<CANopenSubObject subIndex=\"05\" name=\"Motor output voltage Xq\" objectType=\"7\" dataType=\"0003\" lowLimit=\"-32768\" highLimit=\"32767\" accessType=\"rw\" defaultValue=\"0\" PDOmapping=\"TPDO\" />\n\t\t\t\t\t\t<CANopenSubObject subIndex=\"06\" name=\"Sinus output voltage Ua\" objectType=\"7\" dataType=\"0006\" accessType=\"ro\" PDOmapping=\"TPDO\" />\n\t\t\t\t\t\t<CANopenSubObject subIndex=\"07\" name=\"Sinus output voltage Ub\" objectType=\"7\" dataType=\"0006\" accessType=\"ro\" PDOmapping=\"TPDO\" />\n\t\t\t\t\t\t<CANopenSubObject subIndex=\"08\" name=\"Sinus output voltage Uc\" objectType=\"7\" dataType=\"0006\" accessType=\"ro\" PDOmapping=\"TPDO\" />\n\t\t\t\t\t\t<CANopenSubObject subIndex=\"09\" name=\"Sinus output voltage Ud\" objectType=\"7\" dataType=\"0006\" accessType=\"ro\" PDOmapping=\"TPDO\" objFlags=\"00020003\" />\n\t\t\t\t\t</CANopenObject>\n\t\t\t\t\t<CANopenObject index=\"2341\" name=\"Target voltage\" objectType=\"7\" dataType=\"0003\" lowLimit=\"-32768\" highLimit=\"32767\" accessType=\"rw\" defaultValue=\"0\" PDOmapping=\"RPDO\" />\n\t\t\t\t\t<CANopenObject index=\"2342\" name=\"Torque control parameters\" objectType=\"9\" subNumber=\"3\">\n\t\t\t\t\t\t<CANopenSubObject subIndex=\"00\" name=\"Number of entries\" objectType=\"7\" dataType=\"0005\" accessType=\"ro\" defaultValue=\"2\" PDOmapping=\"no\" />\n\t\t\t\t\t\t<CANopenSubObject subIndex=\"01\" name=\"Gain Kpi\" objectType=\"7\" dataType=\"0007\" lowLimit=\"0\" highLimit=\"4294967295\" accessType=\"rw\" PDOmapping=\"no\" />\n\t\t\t\t\t\t<CANopenSubObject subIndex=\"02\" name=\"Integral time Tni\" objectType=\"7\" dataType=\"0006\" lowLimit=\"150\" highLimit=\"2600\" accessType=\"rw\" PDOmapping=\"no\" />\n\t\t\t\t\t</CANopenObject>\n\t\t\t\t\t<CANopenObject index=\"2343\" name=\"Flux control parameters\" objectType=\"9\" subNumber=\"3\">\n\t\t\t\t\t\t<CANopenSubObject subIndex=\"00\" name=\"Number of entries\" objectType=\"7\" dataType=\"0005\" accessType=\"ro\" defaultValue=\"2\" PDOmapping=\"no\" />\n\t\t\t\t\t\t<CANopenSubObject subIndex=\"01\" name=\"Gain Kpi\" objectType=\"7\" dataType=\"0007\" lowLimit=\"0\" highLimit=\"4294967295\" accessType=\"rw\" PDOmapping=\"no\" />\n\t\t\t\t\t\t<CANopenSubObject subIndex=\"02\" name=\"Integral time Tni\" objectType=\"7\" dataType=\"0006\" lowLimit=\"150\" highLimit=\"2600\" accessType=\"rw\" PDOmapping=\"no\" />\n\t\t\t\t\t</CANopenObject>\n\t\t\t\t\t<CANopenObject index=\"2344\" name=\"Velocity control parameters\" objectType=\"9\" subNumber=\"7\">\n\t\t\t\t\t\t<CANopenSubObject subIndex=\"00\" name=\"Number of entries\" objectType=\"7\" dataType=\"0005\" accessType=\"ro\" defaultValue=\"6\" PDOmapping=\"no\" />\n\t\t\t\t\t\t<CANopenSubObject subIndex=\"01\" name=\"Gain KP\" objectType=\"7\" dataType=\"0007\" lowLimit=\"0\" highLimit=\"4294967295\" accessType=\"rw\" PDOmapping=\"RPDO\" />\n\t\t\t\t\t\t<CANopenSubObject subIndex=\"02\" name=\"Integral time TN\" objectType=\"7\" dataType=\"0006\" lowLimit=\"20\" highLimit=\"1000\" accessType=\"rw\" PDOmapping=\"RPDO\" />\n\t\t\t\t\t\t<CANopenSubObject subIndex=\"03\" name=\"Velocity deviation threshold\" objectType=\"7\" dataType=\"0006\" lowLimit=\"0\" highLimit=\"65535\" accessType=\"rw\" defaultValue=\"65535\" PDOmapping=\"RPDO\" objFlags=\"00020000\" />\n\t\t\t\t\t\t<CANopenSubObject subIndex=\"04\" name=\"Velocity deviation time\" objectType=\"7\" dataType=\"0006\" lowLimit=\"1\" highLimit=\"65535\" accessType=\"rw\" defaultValue=\"100\" PDOmapping=\"RPDO\" objFlags=\"00020000\" />\n\t\t\t\t\t\t<CANopenSubObject subIndex=\"05\" name=\"Velocity warning threshold\" objectType=\"7\" dataType=\"0007\" lowLimit=\"1\" highLimit=\"0x007FFFFF\" accessType=\"rw\" defaultValue=\"30000\" PDOmapping=\"RPDO\" objFlags=\"00020000\" />\n\t\t\t\t\t\t<CANopenSubObject subIndex=\"06\" name=\"Integral part option\" objectType=\"7\" dataType=\"0005\" PDOmapping=\"RPDO\" objFlags=\"00020000\" uniqueIDRef=\"UID_PARAM_234406\" />\n\t\t\t\t\t</CANopenObject>\n\t\t\t\t\t<CANopenObject index=\"2345\" name=\"Velocity filter parameters\" objectType=\"9\" subNumber=\"3\">\n\t\t\t\t\t\t<CANopenSubObject subIndex=\"00\" name=\"Number of entries\" objectType=\"7\" dataType=\"0005\" accessType=\"ro\" defaultValue=\"2\" PDOmapping=\"no\" />\n\t\t\t\t\t\t<CANopenSubObject subIndex=\"01\" name=\"Actual velocity filter TF\" objectType=\"7\" dataType=\"0006\" lowLimit=\"0\" highLimit=\"65535\" accessType=\"rw\" PDOmapping=\"RPDO\" objFlags=\"00020000\" />\n\t\t\t\t\t\t<CANopenSubObject subIndex=\"02\" name=\"Display velocity filter\" objectType=\"7\" dataType=\"0006\" lowLimit=\"0\" highLimit=\"65535\" accessType=\"rw\" PDOmapping=\"RPDO\" objFlags=\"00020000\" />\n\t\t\t\t\t</CANopenObject>\n\t\t\t\t\t<CANopenObject index=\"2346\" name=\"Setpoint velocity filter parameters\" objectType=\"9\" subNumber=\"3\">\n\t\t\t\t\t\t<CANopenSubObject subIndex=\"00\" name=\"Number of entries\" objectType=\"7\" dataType=\"0005\" accessType=\"ro\" defaultValue=\"2\" PDOmapping=\"no\" />\n\t\t\t\t\t\t<CANopenSubObject subIndex=\"01\" name=\"Setpoint velocity filter TF\" objectType=\"7\" dataType=\"0006\" lowLimit=\"0\" highLimit=\"65535\" accessType=\"rw\" PDOmapping=\"RPDO\" objFlags=\"00020000\" />\n\t\t\t\t\t\t<CANopenSubObject subIndex=\"02\" name=\"Setpoint filter enable\" objectType=\"7\" dataType=\"0005\" PDOmapping=\"RPDO\" objFlags=\"00020000\" uniqueIDRef=\"UID_PARAM_234602\" />\n\t\t\t\t\t</CANopenObject>\n\t\t\t\t\t<CANopenObject index=\"2347\" name=\"Gain scheduling\" objectType=\"9\" subNumber=\"3\">\n\t\t\t\t\t\t<CANopenSubObject subIndex=\"00\" name=\"Number of entries\" objectType=\"7\" dataType=\"0005\" accessType=\"ro\" defaultValue=\"2\" PDOmapping=\"no\" />\n\t\t\t\t\t\t<CANopenSubObject subIndex=\"01\" name=\"Gain factor Kpn\" objectType=\"7\" dataType=\"0005\" lowLimit=\"0\" highLimit=\"255\" accessType=\"rw\" defaultValue=\"128\" PDOmapping=\"RPDO\" />\n\t\t\t\t\t\t<CANopenSubObject subIndex=\"02\" name=\"Gain factor Kv\" objectType=\"7\" dataType=\"0005\" lowLimit=\"0\" highLimit=\"255\" accessType=\"rw\" defaultValue=\"128\" PDOmapping=\"RPDO\" />\n\t\t\t\t\t</CANopenObject>\n\t\t\t\t\t<CANopenObject index=\"2348\" name=\"Position control parameters\" objectType=\"9\" subNumber=\"2\">\n\t\t\t\t\t\t<CANopenSubObject subIndex=\"00\" name=\"Number of entries\" objectType=\"7\" dataType=\"0005\" accessType=\"ro\" defaultValue=\"1\" PDOmapping=\"no\" />\n\t\t\t\t\t\t<CANopenSubObject subIndex=\"01\" name=\"Gain Kv\" objectType=\"7\" dataType=\"0005\" lowLimit=\"0\" highLimit=\"255\" accessType=\"rw\" PDOmapping=\"RPDO\" />\n\t\t\t\t\t</CANopenObject>\n\t\t\t\t\t<CANopenObject index=\"2349\" name=\"Current feedforward parameters\" objectType=\"9\" subNumber=\"3\">\n\t\t\t\t\t\t<CANopenSubObject subIndex=\"00\" name=\"Number of entries\" objectType=\"7\" dataType=\"0005\" accessType=\"ro\" defaultValue=\"2\" PDOmapping=\"no\" />\n\t\t\t\t\t\t<CANopenSubObject subIndex=\"01\" name=\"Current feedforward factor\" objectT
